vi "Concatenate Array.vi"(1 "process information":dbl[](array[numeric])) -> (0 "concatenated array":dbl[](array[numeric]))   [LabVIEW 2016]
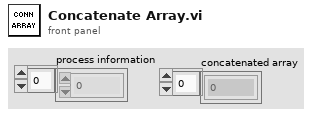
[diagram p1: front panel]
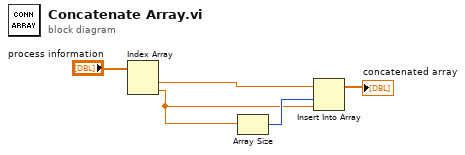
[diagram p0: block diagram]
diagram:
  n1 = Index Array(array="process information") -> (element #1=w2:dbl, element #2=w1:dbl)  [unwired: 2 in]
  n2 = Array Size(array=w1) -> (size(s)=w5:i32)
  n3 = Insert Into Array(array=w2, index=w5, new element=w1) -> (→"concatenated array":dbl[])
